vi "Set-Setpoint.vi"(8 "error in (no error)":errorcluster, 10 "New setpoint / V":dbl min=-5.0 max=5.0, 11 "VISA resource name":refnum<visa-resource-name>) -> (0 "error out":errorcluster, 3 "VISA resource name out":refnum<visa-resource-name>)   [LabVIEW 2014, in "YbTempCtrl.lvlib"]
doc: "Change the setpoint for the lock"
uses:
  YbTempCtrl.lvlib
  Typedefs/OutputChannelTypedef.ctl
panel:
  in  "Output channel":T1
  out "Returned String":string
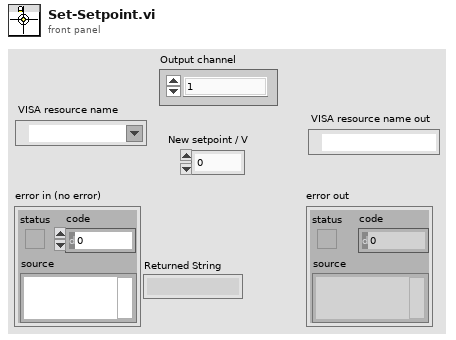
[diagram p1: front panel]
types:
  T1 = typedef "YbTempCtrl.lvlib/OutputChannelTypedef.ctl" = enum16{"1", "2", "3", "4", "BPA", "BPB"}
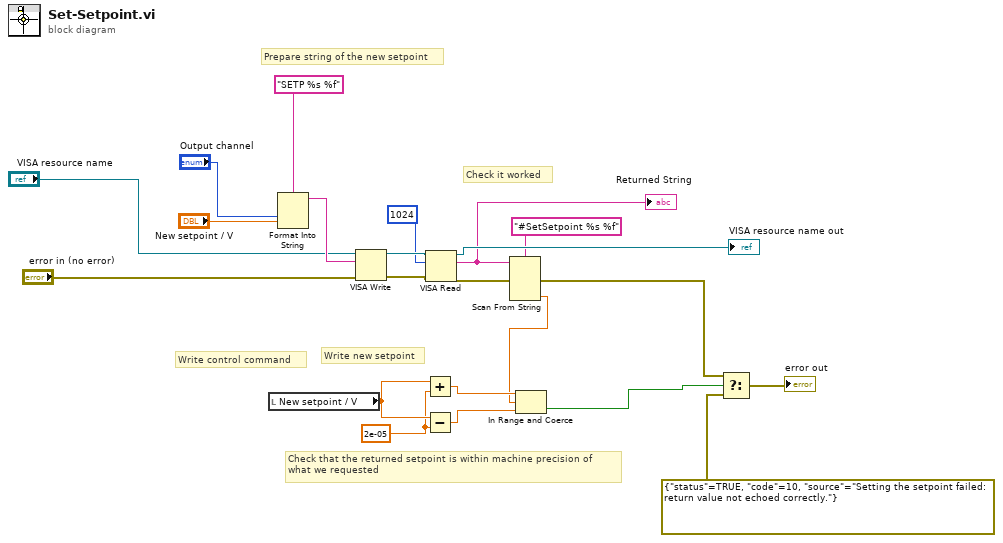
[diagram p0: block diagram]
diagram:
  w19 = 2e-05
  # "Check that the returned setpoint is within machine precision of\nwhat we requested"
  # "Check it worked"
  # "Write new setpoint"
  # "Prepare string of the new setpoint"
  # "Write control command"
  n1 = local read "New setpoint / V"() -> (w20:dbl)
  n2 = Format Into String(format string="SETP %s %f", "Output channel", "New setpoint / V") -> (resulting string=w21:string)  [unwired: 2 in, 1 out]
  n3 = VISA Write(VISA resource name="VISA resource name", write buffer=w21, error in (no error)="error in (no error)") -> (VISA resource name out=w14:refnum<visa-resource-name>, error out=w12:errorcluster)  [unwired: 1 out]
  n4 = Add(x=w20, y=w19) -> (x+y=w18:dbl)
  n5 = Subtract(x=w20, y=w19) -> (x-y=w17:dbl)
  n6 = VISA Read(VISA resource name=w14, byte count=u32 1024, error in (no error)=w12) -> (VISA resource name out=→"VISA resource name out":refnum<visa-resource-name>, read buffer=w10:string, error out=w9:errorcluster)  [unwired: 1 out]
  "Returned String" <- w10
  n7 = Scan From String(format string="#SetSetpoint %s %f", input string=w10, error in=w9) -> (error out=w8:errorcluster, output 2=w2:dbl)  [unwired: 4 in, 2 out]
  n8 = In Range and Coerce(upper limit=w18, x=w2, lower limit=w17) -> (In Range?=w1:bool)  [unwired: 1 out]
  n9 = Select(t=w8, s=w1, f=errorcluster {"status"=TRUE, "code"=10, "source"="Setting the setpoint failed: return value not echoed correctly."}) -> (s? t:f=→"error out":errorcluster)
